vi "Preferences.vi"(11 "Preferences in":T1={"python"="", "arduino CLI"=path "", "pythonCodes"=[], "FontSize"=0, "Text Colors"={"Quote"=46086, "function"=239, "Python"=11817216, "Comment"=15665920, "Triple Quote"=9306312, "Text"=0}, "SSH Logins"=[], "packet size"=32}) -> (0 "error out":errorcluster, 3 "Preferences out":T1={"python"="3.7", "arduino CLI"=path "/Users/crogers/GitHub/ME35_21/PythonIDE/_LVsubs/Arduino/arduino-cli_0.18.3_macOS_64bit", "pythonCodes"=[{"pythonCode"=path "/Users/crogers/Documents/Work/Classes/2021 1Sum/Summer 2021 Codes", "Color"=4060}, {"pythonCode"=path "/Users/crogers/Documents/Work/Classes/2021 1Spr/ME35/MyCodes", "Color"=35136}, {"pythonCode"=path "/Users/crogers/Documents/Current Projects/Python/MicroPythonCodes", "Color"=41416}, {"pythonCode"=path "/Users/crogers/Documents/Python Codes/HiPeaks Code", "Color"=7864500}, {"pythonCode"=path "/Users/crogers/Documents/Current Projects/iRobot Create stuff/ROS2_LV", "Color"=16719872}, {"pythonCode"=path "/Users/crogers/Documents/Work/Classes/2022 1Spr/ME193 - edBots/ME193 Python", "Color"=16747264}], "FontSize"=12, "Text Colors"={"Quote"=46086, "function"=239, "Python"=11817216, "Comment"=16711680, "Triple Quote"=9306312, "Text"=0}, "SSH Logins"=[{"IP Address"="192.168.1.20", "Username"="pi", "password"="password"}], "packet size"=32})   [LabVIEW 2022 SP3]
uses:
  Preferences.ctl
  <vilib>/Utility/error.llb/Trim Whitespace One-Sided.vi
  ColorText/Color_Globals.vi
panel:
  out "text":string
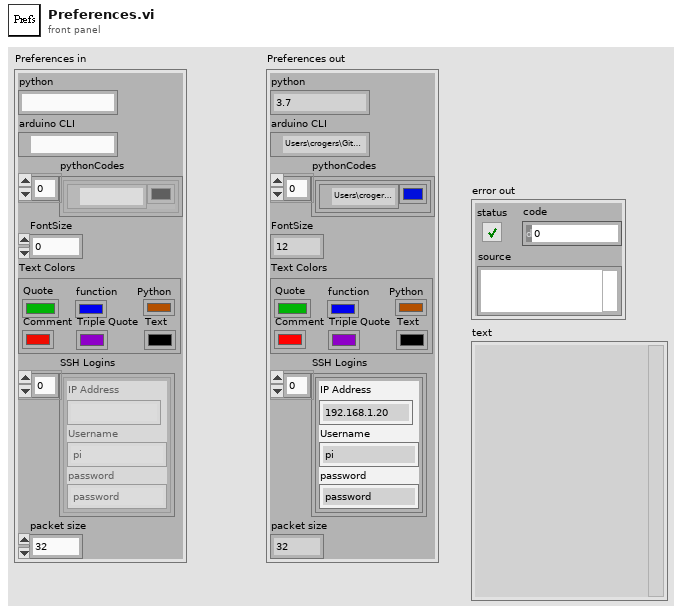
[diagram p1: front panel]
types:
  T1 = typedef "Preferences.ctl" = cluster{"python":string, "arduino CLI":path, "pythonCodes":cluster{"pythonCode":path, "Color":u32}[], "FontSize":u8, "Text Colors":cluster{"Quote":u32, "function":u32, "Python":u32, "Comment":u32, "Triple Quote":u32, "Text":u32}, "SSH Logins":cluster{"IP Address":string, "Username":string, "password":string}[], "packet size":u8}
  T2 = cluster{"IP Address":string, "Username":string, "password":string}[]
  T3 = cluster{"python":string, "arduinoCLI":string, "PythonCodePath":string, "FontSize":string, "Colors":string, "Ssh Logins":string, "packet size":string}
  T4 = cluster{"Quote":u32, "function":u32, "Python":u32, "Comment":u32, "Triple Quote":u32, "Text":u32}
  T5 = cluster{"[0]":string, "[1]":string, "[2]":string, "[3]":string, "[4]":string, "[5]":string, "[6]":string}
  T6 = cluster{"array[0]":u32, "array[1]":u32, "array[2]":u32, "array[3]":u32, "array[4]":u32, "array[5]":u32}
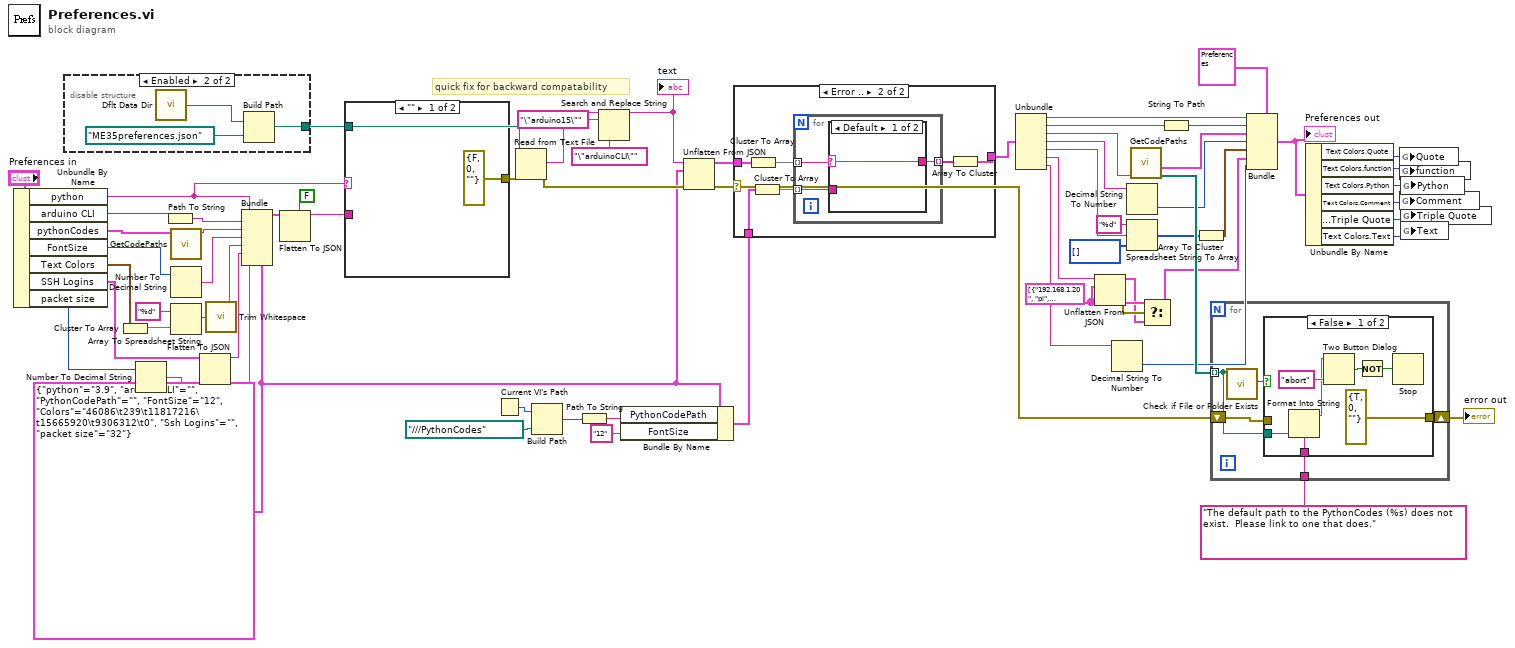
[diagram p0: block diagram]
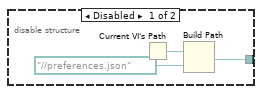
[diagram p2: hidden frame]
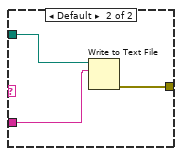
[diagram p4: hidden frame]
diagram:
  w7 = T2 [{"IP Address"="192.168.1.20", "Username"="pi", "password"="password"}] ("SSH Logins")
  w47 = T3 {"python"="3.9", "arduinoCLI"="", "PythonCodePath"="", "FontSize"="12", "Colors"="46086\t239\t11817216\t15665920\t9306312\t0", "Ssh Logins"="", "packet size"="32"} ("Preferences")
  # "quick fix for backward compatability"
  n1 = Unbundle By Name("Preferences in") -> ("python"=w63:string, "arduino CLI"=w62:path, "pythonCodes"=w55:cluster{"pythonCode":path, "Color":u32}[], "FontSize"=w44:u8, "Text Colors"=w37:T4, "SSH Logins"=w11:T2, "packet size"=w3:u8)
  n2 = disable-structure shown="Enabled" {
    disable-tunnel: [w68 w71] -> w58
    frame Disabled {
      n3 = Current VI's Path() -> (path=w70:path)
      n4 = Build Path(base path=w70, name or relative path=path "../../preferences.json") -> (appended path=w68:path)
    }
    frame Enabled {
      n5 = call <vilib>:"Dflt Data Dir.vi"() -> ("App:Default Data Directory"=w73:path)
      n6 = Build Path(base path=w73, name or relative path=path "ME35preferences.json") -> (appended path=w71:path)
    }
  }
  n7 = Cluster To Array(cluster=w37) -> (array=w34:u32[])
  n8 = Number To Decimal String(number=w3) -> (decimal integer string=w2:string)  [unwired: 1 in]
  n9 = Path To String(path=w62) -> (string=w57:string)
  n10 = call "GetCodePaths.vi"("pythonCodes"=w55) -> ("stringOut"=w56:string)  [unwired: 8 in, 2 out]
  n11 = Number To Decimal String(number=w44) -> (decimal integer string=w43:string)  [unwired: 1 in]
  n12 = Array To Spreadsheet String(array=w34, 3:"%d" ("format string")) -> (spreadsheet string=w35:string)  [unwired: 1 in]
  n13 = Flatten To JSON(anything=w11) -> (JSON string=w10:string)  [unwired: 2 in, 1 out]
  n14 = call <vilib>:"Trim Whitespace.vi"("string"=w35) -> ("trimmed string"=w30:string)  [unwired: 1 in]
  n15 = Bundle(cluster=w47, "python"=w63, "arduinoCLI"=w57, "PythonCodePath"=w56, "FontSize"=w43, "Colors"=w30, "Ssh Logins"=w10, "packet size"=w2) -> (w60:T3)
  n16 = Flatten To JSON(enable LabVIEW extensions? (T)=FALSE, anything=w60) -> (JSON string=w59:string)  [unwired: 1 in, 1 out]
  n17 = case shown="\"\"" w63 {
    tunnel: [errorcluster {"status"=FALSE, "code"=0, "source"=""} ("error out") w77] -> w65
    tunnel: w58 -> [_ w76]
    tunnel: w59 -> [_ w75]
    frame "" {
    }
    frame Default {
      n18 = Write to Text File(file (use dialog)=w76, text=w75) -> (error out=w77:errorcluster)  [unwired: 2 in, 2 out]
    }
  }
  n19 = Current VI's Path() -> (path=w50:path)
  n20 = Read from Text File(file (use dialog)=w58, error in=w65) -> (text=w13:string, error out=w66:errorcluster)  [unwired: 2 in, 2 out]
  n21 = Build Path(base path=w50, name or relative path=path "../../../PythonCodes") -> (appended path=w42:path)
  n22 = Path To String(path=w42) -> (string=w48:string)
  n23 = Search and Replace String(input string=w13, search string="\"arduino15\"", replace string="\"arduinoCLI\"" ("search string")) -> (result string=w12:string)  [unwired: 5 in, 3 out]
  "text" <- w12
  n24 = Bundle By Name(cluster=w47, "PythonCodePath"=w48, "FontSize"="12") -> (w46:T3)
  n25 = Unflatten From JSON(JSON string=w12, type and defaults=w47, error in (no error)=w66) -> (value=w67:T3, error out=w41:errorcluster)  [unwired: 4 in]
  n26 = case shown="Error .." w41 {
    tunnel: w67 -> [w78 w84]
    tunnel: [w78 w81] -> w51
    tunnel: w46 -> [_ w80]
    frame No Error {
    }
    frame Error {
      n27 = Cluster To Array(cluster=w84) -> (array=w83:string[])
      n28 = Cluster To Array(cluster=w80) -> (array=w79:string[])
      n29 = for {
        tunnel: w83 -> [w87] mode=indexing
        tunnel: [w86] -> w82 mode=indexing
        tunnel: w79 -> [w85] mode=indexing
        n30 = case shown="Default" w87 {
          selector: w87 -> [w88 _]
          tunnel: [w88 w89] -> w86
          tunnel: w85 -> [_ w89]
          frame Default {
          }
          frame "" {
          }
        }
      }
      n31 = Array To Cluster(array=w82) -> (cluster=w81:T5)
    }
  }
  n32 = Unbundle(w51) -> ("[0]"=w53:string, "[1]"=w52:string, "[2]"=w18:string, "[3]"=w17:string, "[4]"=w16:string, "[5]"=w9:string, "[6]"=w4:string)
  n33 = Unflatten From JSON(JSON string=w9, type and defaults=w7) -> (value=w6:T2, error out=w8:errorcluster)  [unwired: 5 in]
  n34 = Decimal String To Number(string=w4) -> (number=w1:i32)  [unwired: 2 in, 1 out]
  n35 = Decimal String To Number(string=w17) -> (number=w20:i32)  [unwired: 2 in, 1 out]
  n36 = Spreadsheet String To Array(format string="%d", spreadsheet string=w16, array type (2D Dbl)=u32[] [] ("array")) -> (array=w32:u32[])  [unwired: 1 in]
  n37 = call "GetCodePaths.vi"("stringIn"=w18) -> ("Paths out"=w38:path[], "pythonCodes out"=w21:cluster{"pythonCode":path, "Color":u32}[])  [unwired: 8 in, 1 out]
  n38 = Select(t=w7, s=w8, f=w6) -> (s? t:f=w5:T2)
  n39 = String To Path(string=w52) -> (path=w54:path)
  n40 = Array To Cluster(array=w32) -> (cluster=w19:T6)
  n41 = for {
    tunnel: "The default path to the PythonCodes (%s) does not exist.  Please link to one that does." ("message") -> [w91]
    shift-right: [w92] -> w40
    shift-left: w41 -> [w93]
    tunnel: w38 -> [w90] mode=indexing
    n42 = call <vilib>:"Check if File or Folder Exists.vi"("path"=w90) -> ("file or folder exists?"=w94:bool)  [unwired: 8 in, 2 out]
    n43 = case shown="False" w94 {
      tunnel: w93 -> [_ w102]
      tunnel: [errorcluster {"status"=TRUE, "code"=0, "source"=""} ("error out") w102] -> w92
      tunnel: w91 -> [w97 _]
      tunnel: w90 -> [w95 _]
      frame False {
        n44 = Format Into String(format string=w97, w95) -> (resulting string=w96:string)  [unwired: 2 in, 1 out]
        n45 = Two Button Dialog(message=w96, 1:"abort" ("F button name (\"Cancel\")")) -> (T button?=w99:bool)  [unwired: 1 in]
        n46 = Not(x=w99) -> (.not. x?=w98:bool)
        n47 = Stop(stop? (T)=w98) -> ()
      }
      frame True {
      }
    }
  }
  "error out" <- w40
  n48 = Bundle(cluster=T1 {"python"="3.7", "arduino CLI"=path "/Applications/Arduino.app", "pythonCodes"=[{"pythonCode"=path "/Users/crogers/Desktop/Summer2021/PythonCodes", "Color"=0}, {"pythonCode"=path "/Users/crogers/Documents/Work/Classes/2021 1Spr/ME35/MyCodes", "Color"=35136}, {"pythonCode"=path "/Users/crogers/Documents/Python Codes/HiPeaks Code", "Color"=7864500}, {"pythonCode"=path "/Users/crogers/GitHub/ME35_21/PythonCodes", "Color"=10421504}], "FontSize"=12, "Text Colors"={"Quote"=46086, "function"=239, "Python"=11817216, "Comment"=15665920, "Triple Quote"=9306312, "Text"=0}, "SSH Logins"=[], "packet size"=32} ("Preferences in"), "python"=w53, "arduino CLI"=w54, "pythonCodes"=w21, "FontSize"=w20, "Text Colors"=w19, "SSH Logins"=w5, "packet size"=w1) -> (w29:T1)
  "Preferences out" <- w29
  n49 = Unbundle By Name(w29) -> ("Text Colors.Quote"=w22:u32, "Text Colors.function"=w23:u32, "Text Colors.Python"=w24:u32, "Text Colors.Comment"=w25:u32, "Text Colors.Triple Quote"=w26:u32, "Text Colors.Text"=w27:u32)
  n50 = global write "Color_Globals.vi" "Quote"(w22) -> ()
  n51 = global write "Color_Globals.vi" "function"(w23) -> ()
  n52 = global write "Color_Globals.vi" "Comment"(w25) -> ()
  n53 = global write "Color_Globals.vi" "Python"(w24) -> ()
  n54 = global write "Color_Globals.vi" "Triple Quote"(w26) -> ()
  n55 = global write "Color_Globals.vi" "Text"(w27) -> ()
